vi "Do.vi"(8 "error in (no error)":errorcluster, 10 "Actor in":refnum<class "Actor.lvclass">, 11 "Iteration Msg":refnum<class "Abstract Iteration Msg.lvclass">) -> (0 "error out":errorcluster, 2 "Actor out":refnum<class "Actor.lvclass">)   [LabVIEW 2023, in "Iterator Actor.lvlib" / "Abstract Iteration Msg.lvclass"]
doc: "(<B>Filename</B>: Actor Framework.lvlib:Message.lvclass:Do.vi)\n\nDefines what a message does when it is received by an actor. Generally, a message instructs an actor to invoke one of its methods. By default, this method does nothing. A child class must override it to define behavior."
uses:
  Abstract Iteration Msg.lvclass
  <vilib>/ActorFramework/Actor/Actor.lvclass
  Abstract Iteration Msg.lvclass/Abstract Iteration Msg.ctl
  Notify Iteration Msg/Notify Iteration Msg.lvclass
  <userlib>/_OpenG.lib/error/error.llb/openg_error.lvlib
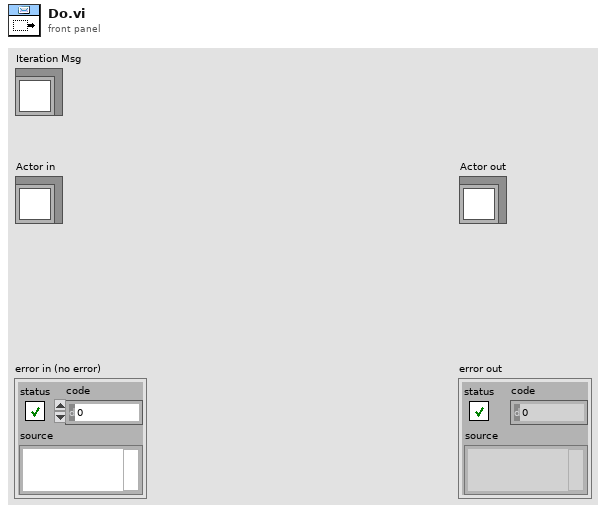
[diagram p1: front panel]
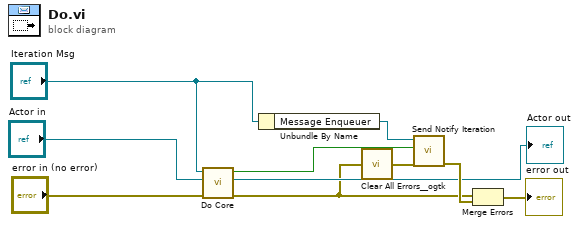
[diagram p0: block diagram]
diagram:
  n1 = call-dynamic "Do Core.vi"("error in (no error)"="error in (no error)", "Actor in"="Actor in", "Message in"="Iteration Msg") -> ("error out"=w1:errorcluster, "Actor out"=→"Actor out":refnum<class "Actor.lvclass">, "Iterate"=w3:bool)  [unwired: 6 in]
  n2 = Unbundle By Name("Iteration Msg") -> ("Message Enqueuer"=w10:refnum<class "Message Enqueuer.lvclass">)
  n3 = call <userlib>:"Clear All Errors__ogtk.vi"("Error In"=w1) -> ("Error Out"=w2:errorcluster)  [unwired: 3 in]
  n4 = call "Send Notify Iteration.vi"("error in (no error)"=w2, "Iterate (T)"=w3, "Message Enqueuer in"=w10) -> ("error out"=w9:errorcluster)  [unwired: 7 in, 1 out]
  n5 = Merge Errors(w1, w9) -> (→"error out":errorcluster)
